vi "Get Main.Parmeters.vi"(0 "Main":string="0", 1 "VI Ref":refnum<vi>, 9 "VariableName":string, 11 "error in (no error)":errorcluster, 12 "Alarm":bool=TRUE) -> (2 "string":string, 3 "Unit":string, 4 "DBL Value":dbl, 6 "Value":string, 10 "Boolean":bool, 13 "Full Results":string[][](array[string]), 14 "Results":string[](array[string]), 15 "error out":errorcluster)   [LabVIEW 2017, in "SQLite.lvclass"]
doc: "get Parmeters.\n2015-11-03 10:59:46\n蒋松\njiangsong@outlook.com"
uses:
  SQLite.lvclass
  SQLiteFileName.ctl
  TabelFullName.ctl
  <userlib>/LabSQL/LabSQL.lvlib
  <userlib>/sushu/sushu.lvlib
panel:
  out "number (0 to 1)":dbl
  out "Select SQL CMD":string
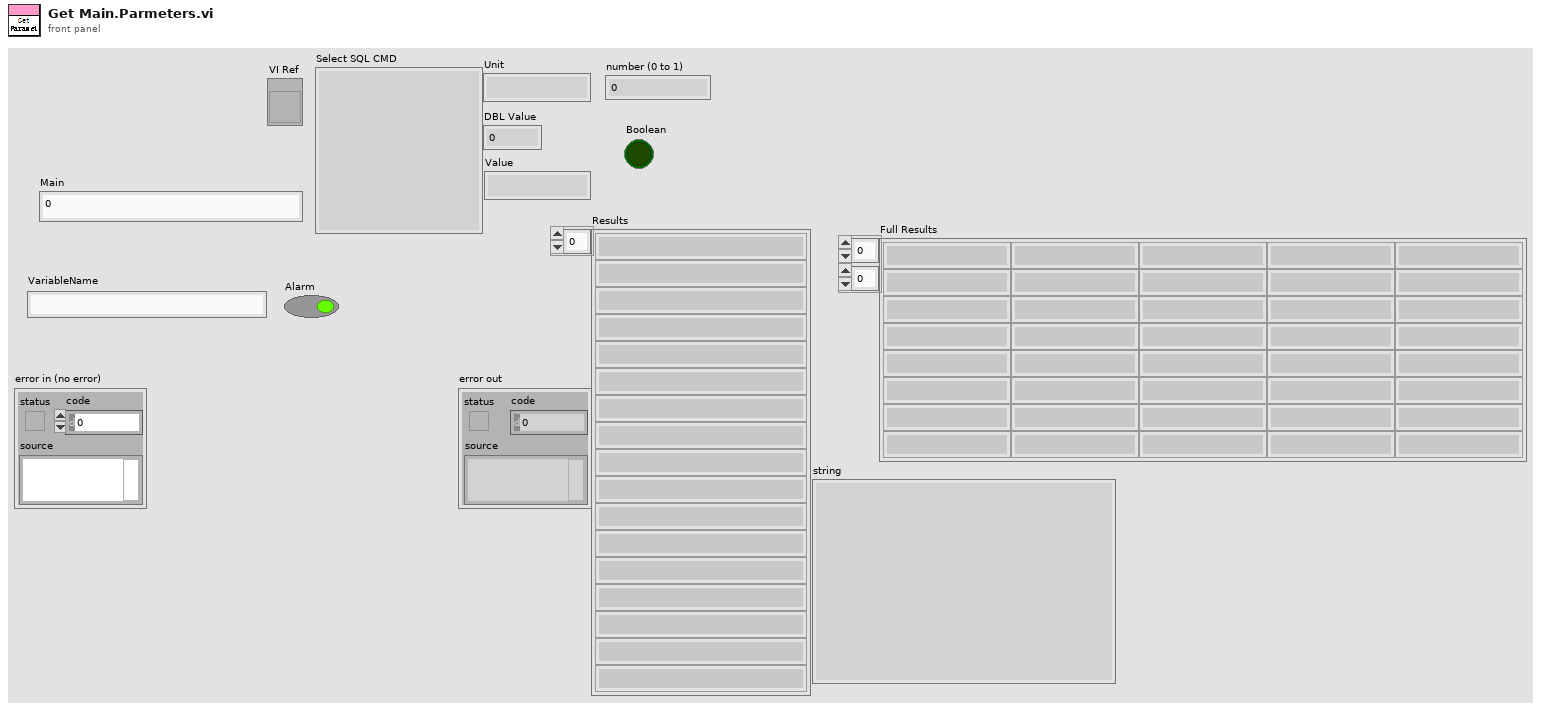
[diagram p1: front panel]
types:
  T1 = enum16{"Initialize", "Read", "Write", "UnInitialize"}
  T2 = typedef "SQLite.lvclass/TabelFullName.ctl" = string
  T3 = typedef "SQLite.lvclass/SQLiteFileName.ctl" = string
  T4 = cluster{"Current VI Reference":refnum<vi>, "Close Panel on Exit?":bool}
  T5 = cluster{"Core":cluster{"Current VI Reference":refnum<vi>, "Close Panel on Exit?":bool}, "VI Name":string}
  T6 = enum16{"Other", "SQL2008", "SQLite", "Access", "MySQL"}
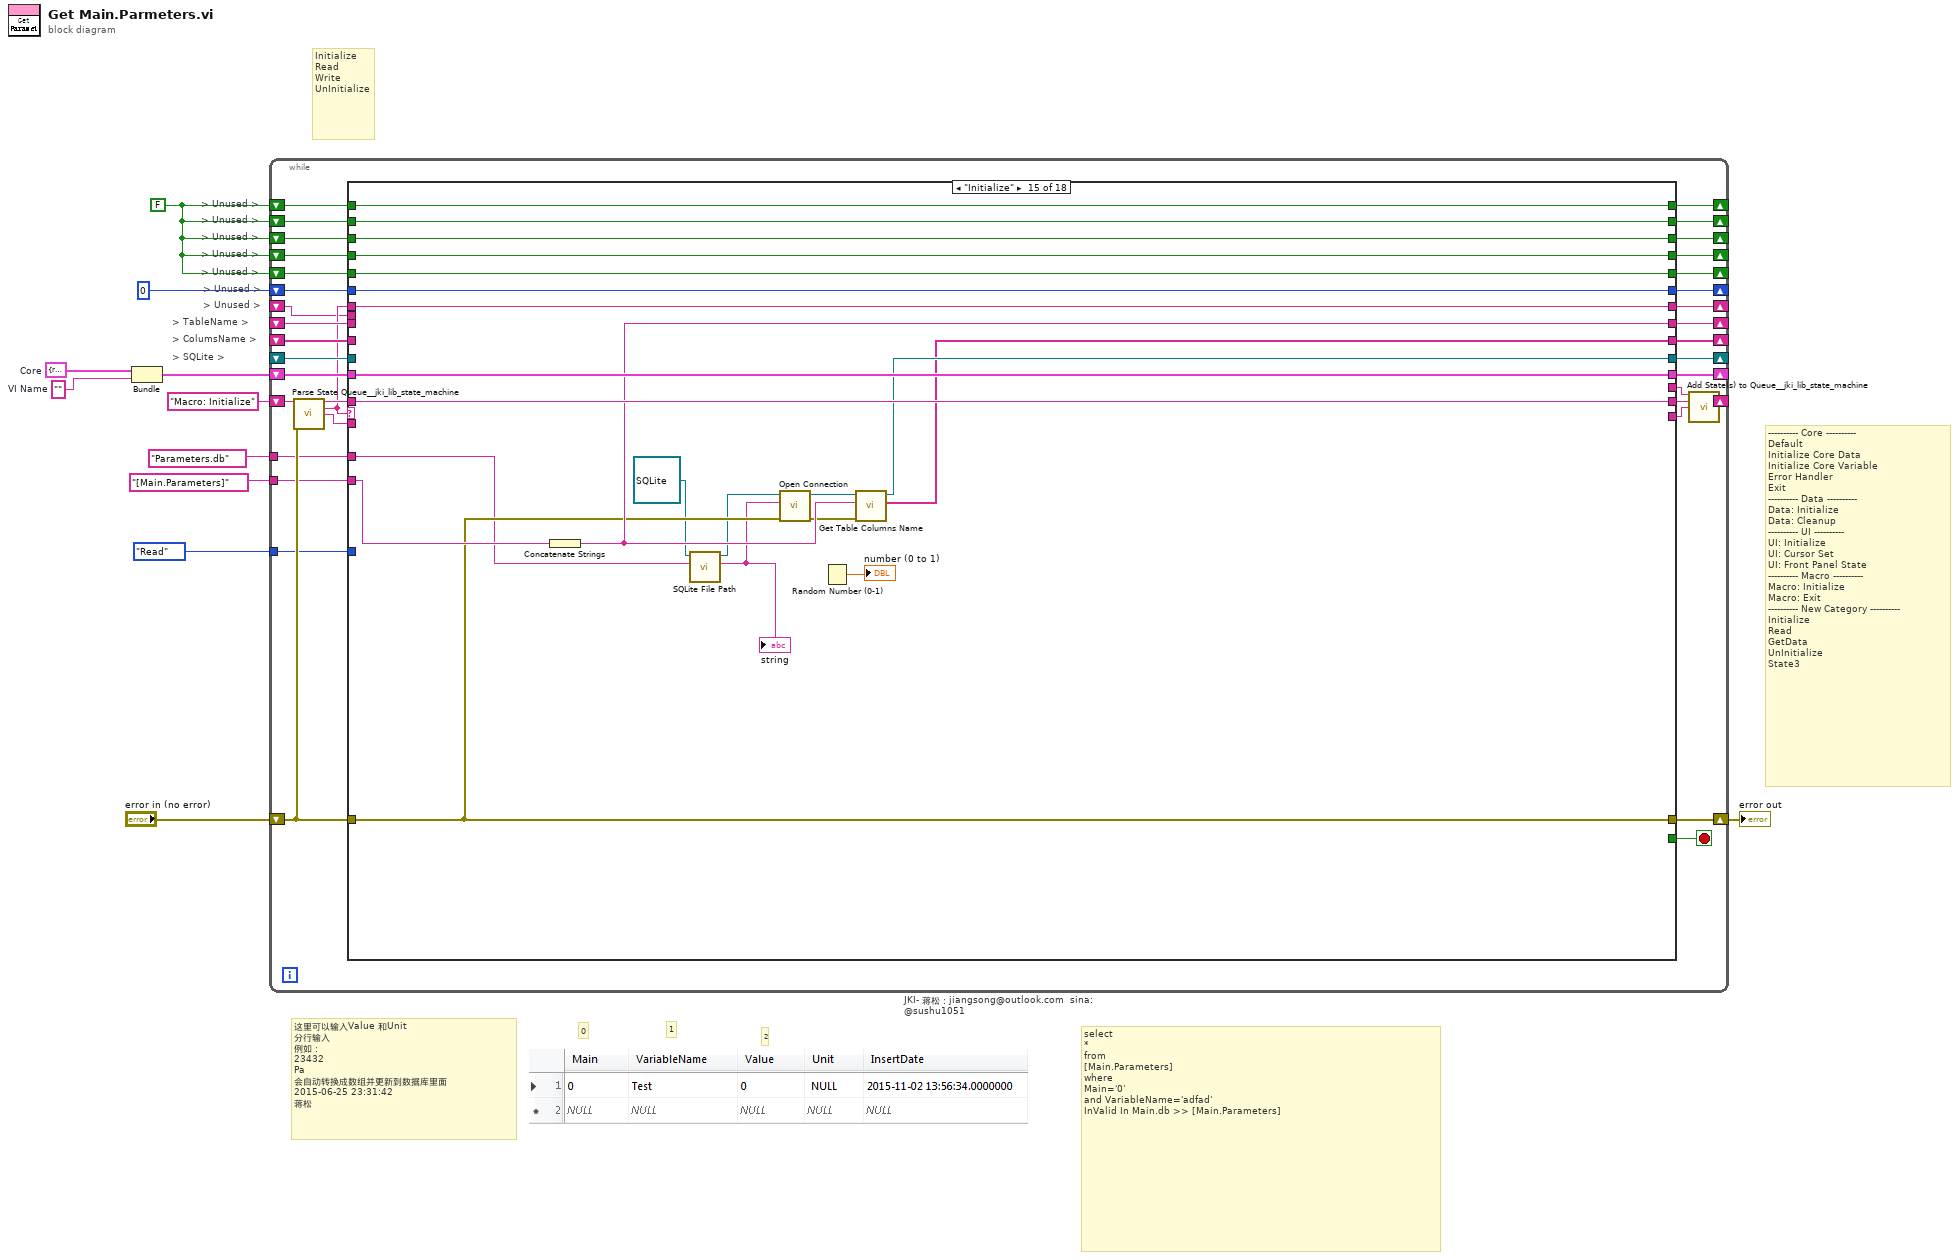
[diagram p0: block diagram]
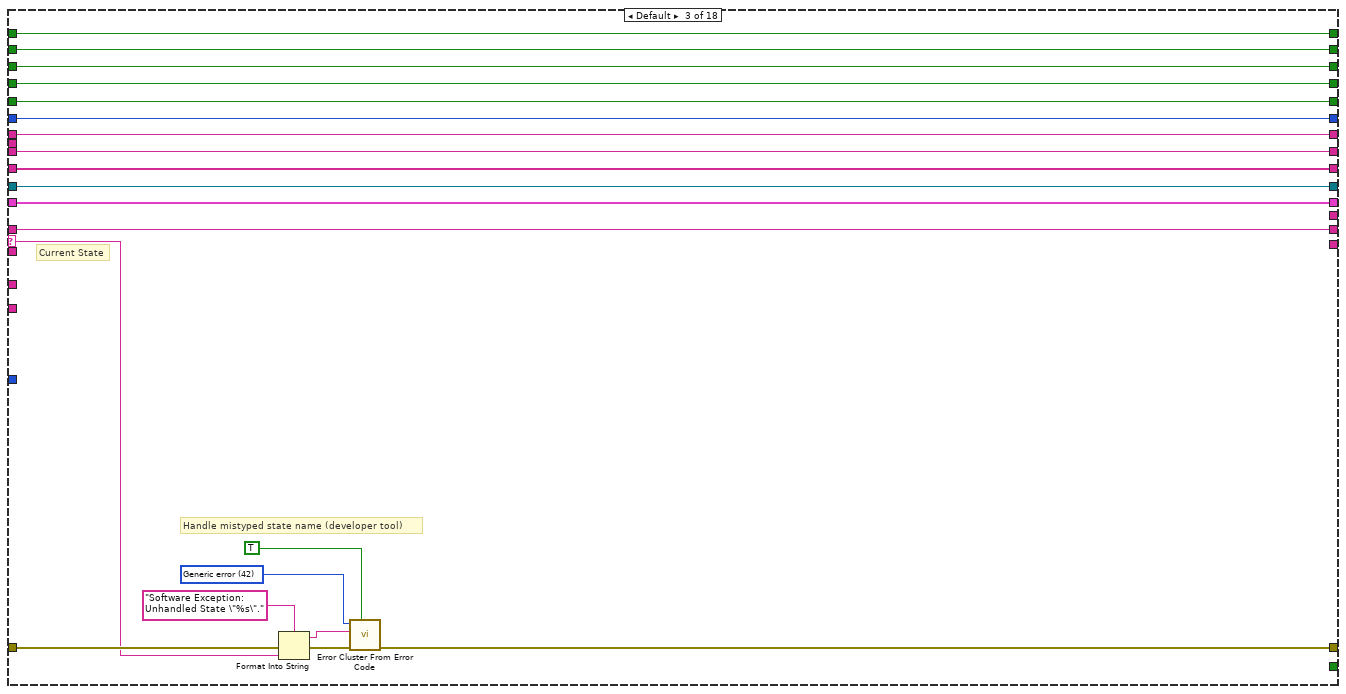
[diagram p4: hidden frame]
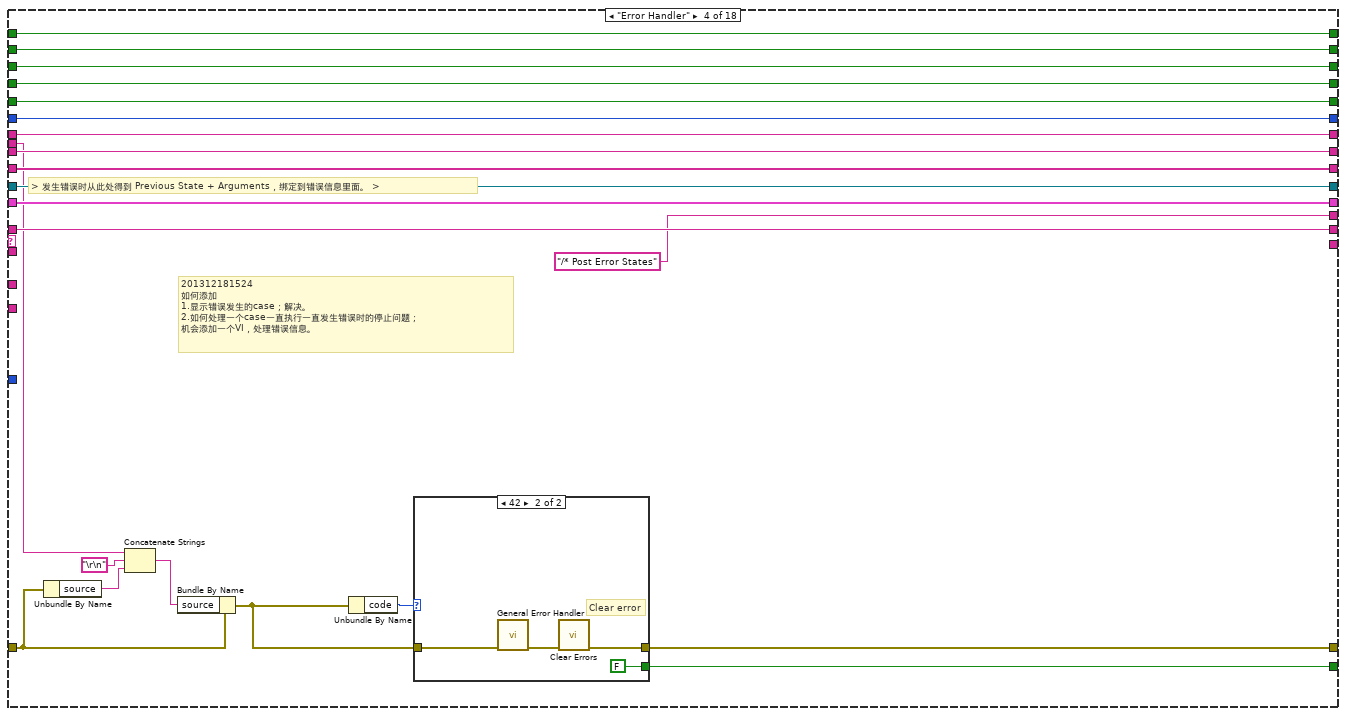
[diagram p5: hidden frame]
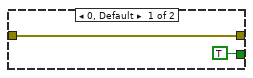
[diagram p6: hidden frame]
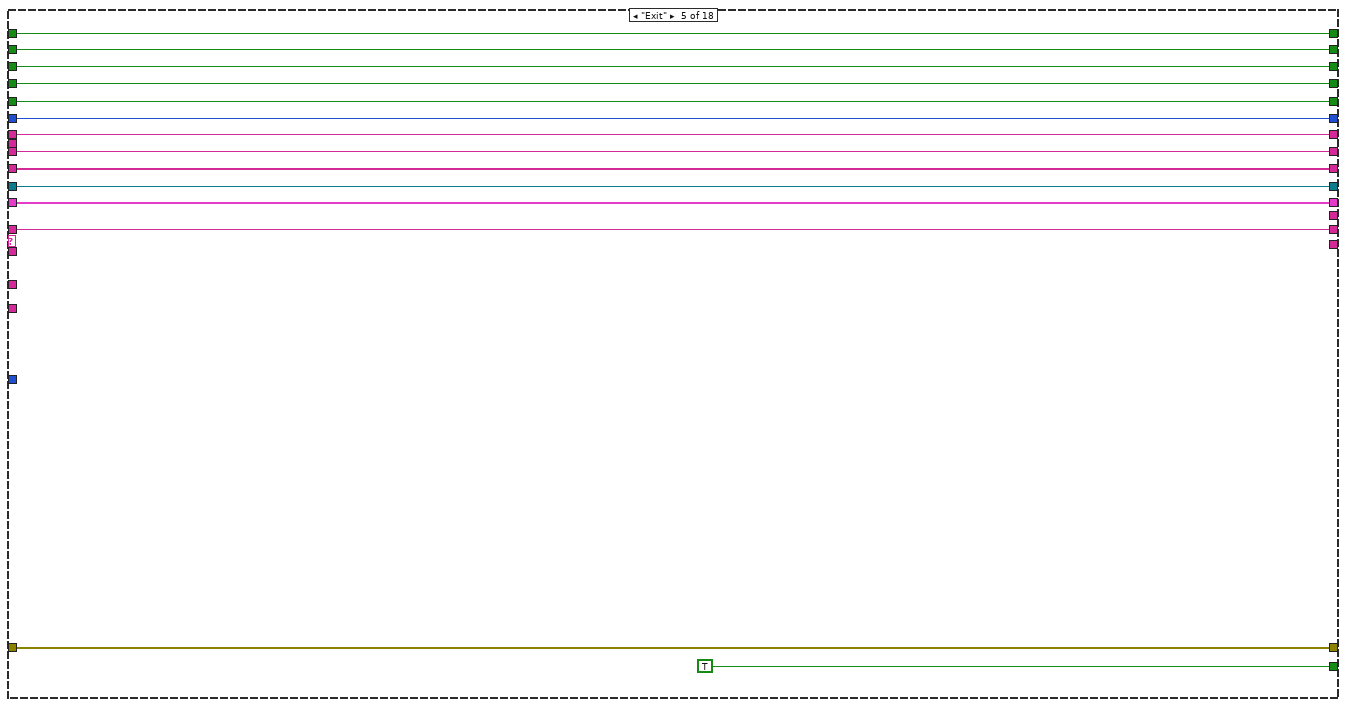
[diagram p7: hidden frame]
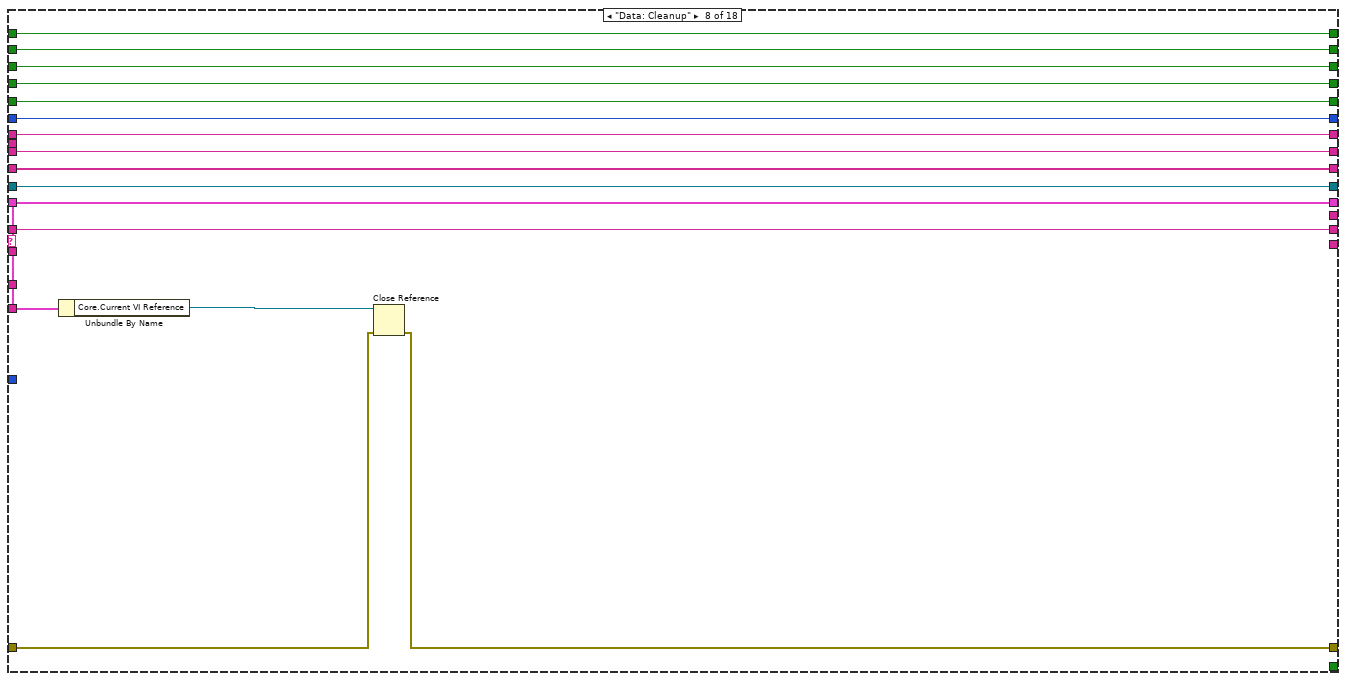
[diagram p10: hidden frame]
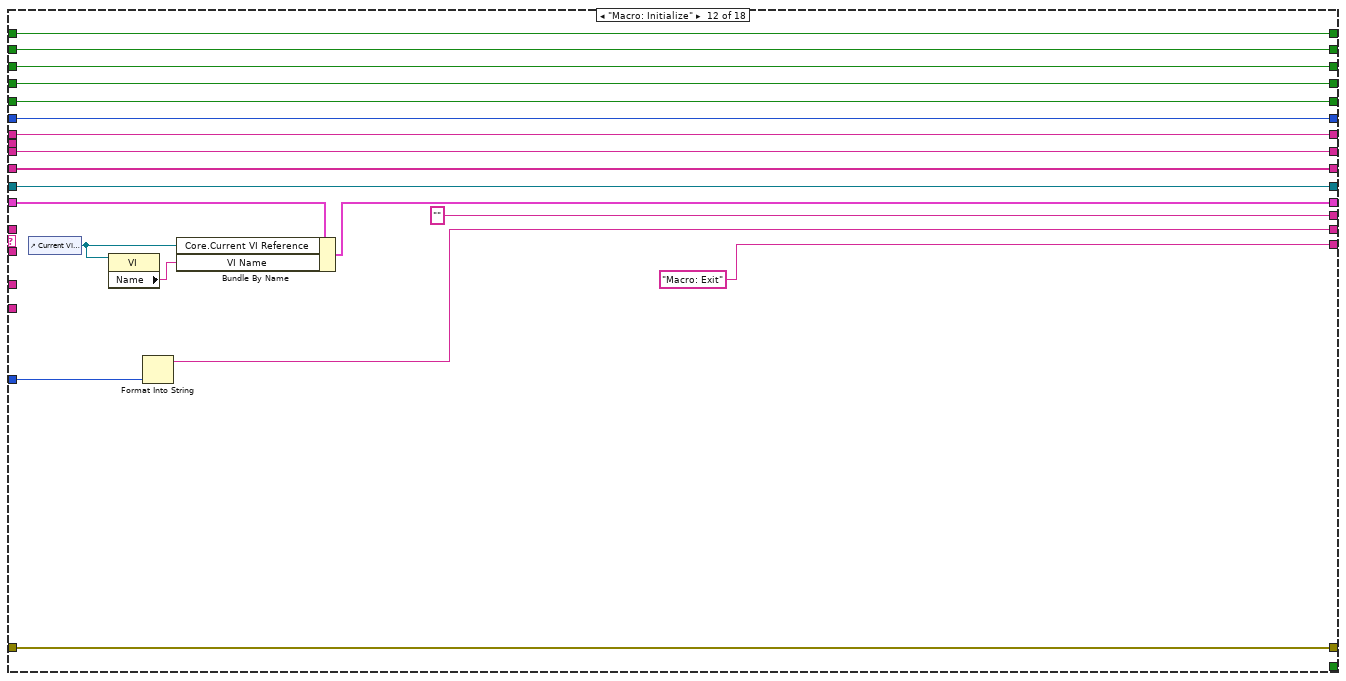
[diagram p14: hidden frame]
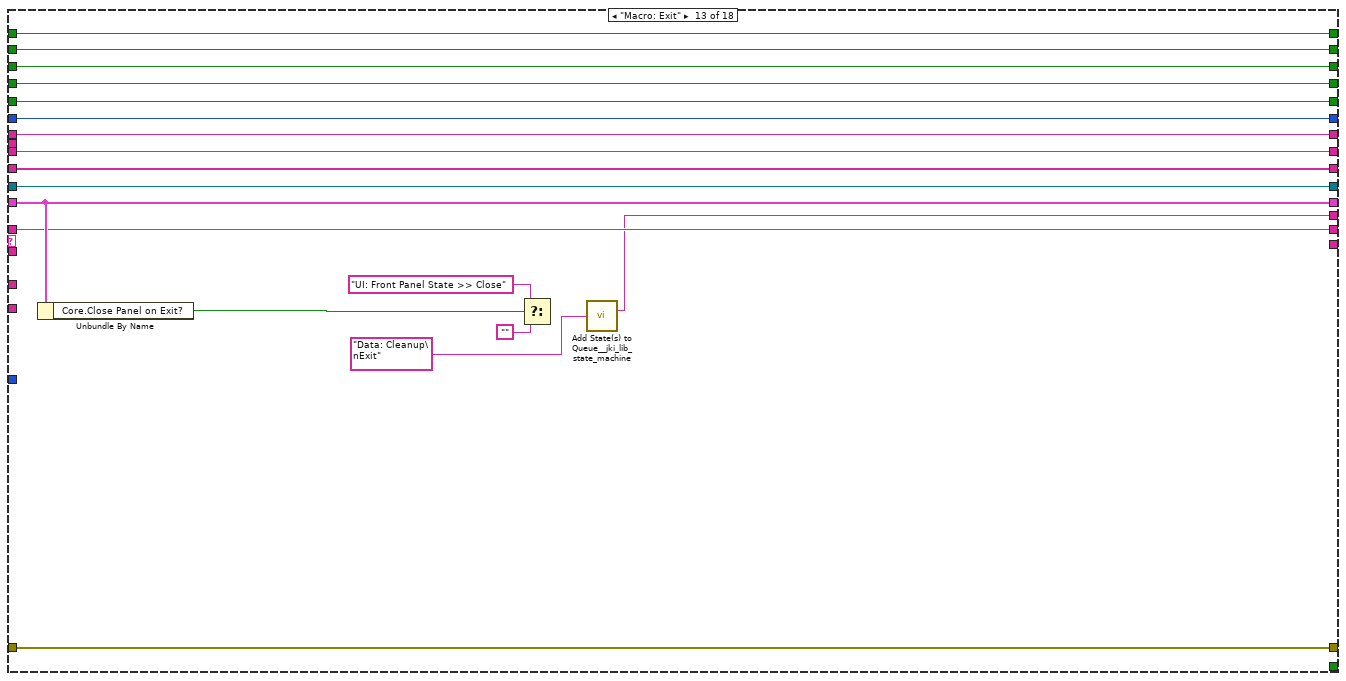
[diagram p15: hidden frame]
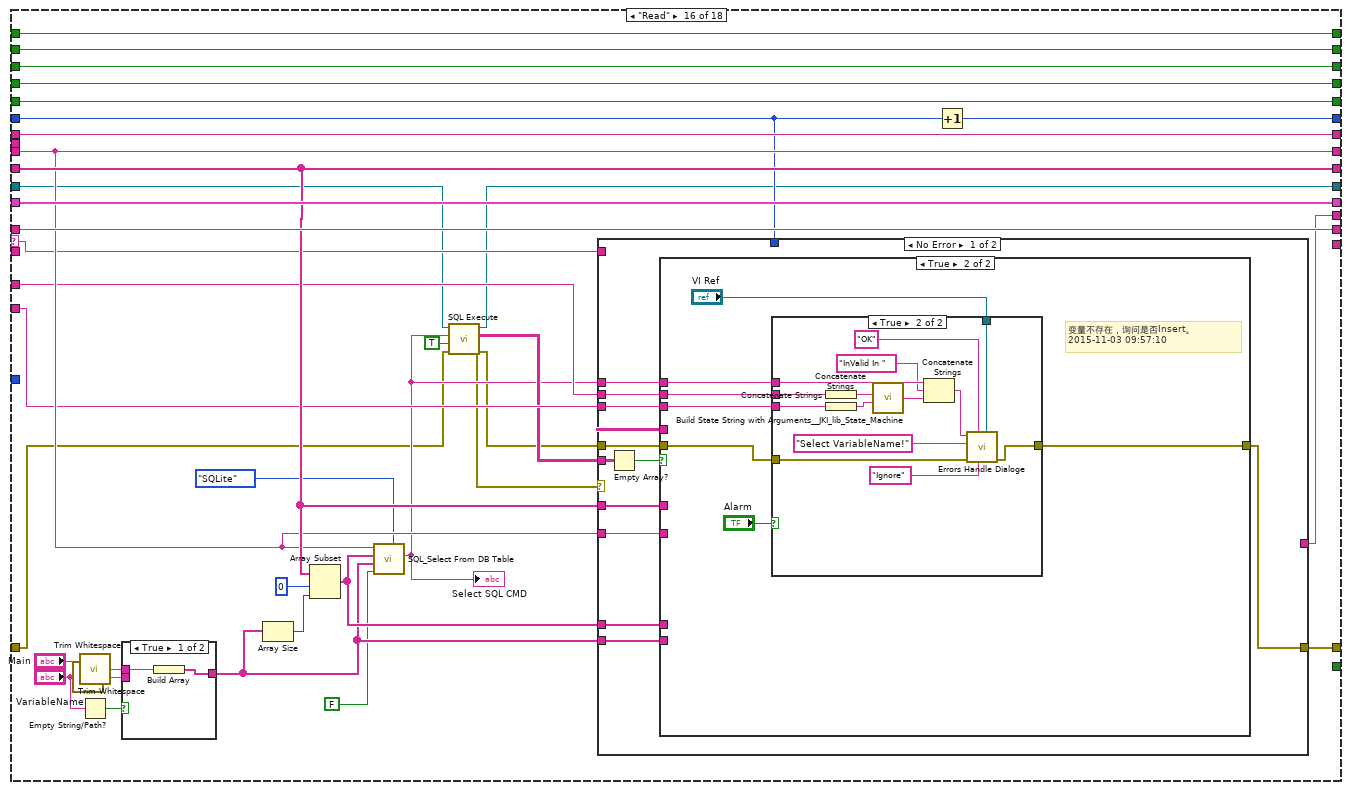
[diagram p17: hidden frame]
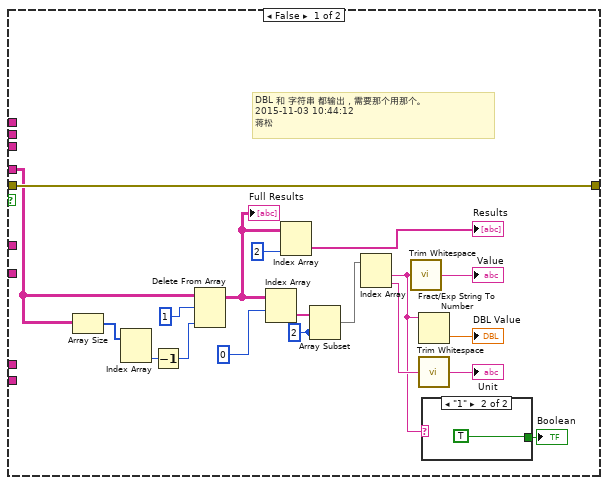
[diagram p18: hidden frame]
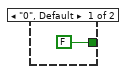
[diagram p19: hidden frame]
diagram:
  w11 = ""  # VI Name
  w10 = T4 {"Current VI Reference"=refnum, "Close Panel on Exit?"=FALSE}  # Core
  w6 = FALSE
  # "Initialize\nRead\nWrite\nUnInitialize"
  # "> Unused >"
  # "> Unused >"
  # "> Unused >"
  # "> Unused >"
  # "> Unused >"
  # "> Unused >"
  # "> SQLite >"
  # "> ColumsName >"
  # "> TableName >"
  # "> Unused >"
  # "---------- Core ----------\nDefault\nInitialize Core Data\nInitialize Core Variable\nError Handler\nExit\n---------- Data ----------\nData: Initialize\nData: Cleanup\n---------- UI ----------\nUI: Initialize\nUI: Cursor Set\nUI: Front Panel State\n---------- Macro ----------\nMacro: Initialize\nMacro: Exit\n---------- New Category ----------\nInitialize\nRead\nGetData\nUnInitialize\nState3"
  # "select\n*\nfrom\n[Main.Parameters]\nwhere\nMain='0'\nand VariableName='adfad'\nInValid In Main.db >> [Main.Parameters]"
  # "2"
  # "1"
  # "0"
  # "这里可以输入Value 和Unit\n分行输入\n例如：\n23432\nPa\n会自动转换成数组并更新到数据库里面\n2015-06-25 23:31:42\n蒋松"
  n1 = Bundle("Core"=w10, "VI Name"=w11) -> (w9:T5)  [unwired: 1 in]
  n2 = while "JKI- 蒋松：jiangsong@outlook.com  sina: @sushu1051" {
    shift-right: [w45] -> w3
    shift-left: "error in (no error)" -> [w43]
    shift-right: [w33] -> _
    shift-left: "Macro: Initialize" -> [w34]
    shift-right: [w40] -> _
    shift-left: _ -> [w42]
    shift-right: [w41] -> _
    shift-left: _ -> [w12]
    shift-right: [w35] -> _
    shift-left: w9 -> [w38]
    shift-right: [w36] -> _
    shift-left: _ -> [w29]
    shift-right: [w37] -> _
    shift-left: _ -> [w39]
    shift-right: [w28] -> _
    shift-left: 0 -> [w27]
    shift-right: [w20] -> _
    shift-left: w6 -> [w18]
    shift-right: [w19] -> _
    shift-left: w6 -> [w17]
    shift-right: [w23] -> _
    shift-left: w6 -> [w24]
    shift-right: [w22] -> _
    shift-left: w6 -> [w21]
    shift-right: [w25] -> _
    shift-left: w6 -> [w26]
    tunnel: T1."Read" ("CMD") -> [w16]
    tunnel: T3 "Parameters.db" ("SQLiteFileName") -> [w15]
    tunnel: T2 "[Main.Parameters]" ("TabelFullName") -> [w14]
    stop <- w44 stop-if-true
    n3 = call <vilib>:"Parse State Queue__jki_lib_state_machine.vi"("State Queue"=w34, "Error In (no error)"=w43) -> ("Remaining States"=w47:string, "Current State"=w13:string, "Arguments"=w46:string)  [unwired: 10 in, 1 out]
    n4 = case shown="\"Initialize\"" w13 {
      selector: w13 -> [_ _ w81 _ _ _ _ _ _ _ _ _ _ _ _ w299 _ _]
      tunnel: w47 -> [w60 w67 w80 w107 w128 w142 w156 w168 w183 w196 w209 _ w242 w259 w286 w321 w405 w420]
      tunnel: w46 -> [_ _ _ _ _ _ _ _ _ _ _ _ _ _ _ _ _ _]
      tunnel: [w59 w73 w82 w101 w130 w144 w158 w170 w185 w198 w211 w231 w249 w262 w271 w300 w393 w406] -> w45
      tunnel: w43 -> [w59 w73 w83 w111 w130 w144 w158 w171 w185 w198 w211 w231 w249 w262 w271 w292 w393 w407]
      tunnel: [w60 w67 w80 w107 w128 w142 w156 w168 w183 w196 w209 w217 w242 w259 w286 w321 w405 w420] -> w32
      tunnel: [_ _ _ w100 TRUE _ _ _ _ _ _ _ _ _ _ _ _ _] -> w44
      tunnel: w13 -> [w58 w72 w93 w115 w135 w148 w161 w176 w189 w202 w215 w234 w252 w265 w285 w301 w395 w419]
      tunnel: w42 -> [w57 w71 w92 w114 w134 w147 w160 w175 w188 w201 w214 w233 w251 w264 _ w305 w404 w418]
      tunnel: [w58 w72 w93 w115 w135 w148 w161 w176 w189 w202 w215 w234 w252 w265 w285 w301 w395 w419] -> w41
      tunnel: [w57 w71 w92 w114 w134 w147 w160 w175 w188 w201 w214 w233 w251 w264 w273 w305 w404 w418] -> w40
      tunnel: w39 -> [w56 w70 w91 w113 w133 w146 w159 w174 w187 w200 w213 w232 w250 w263 _ w306 w403 w417]
      tunnel: w29 -> [w54 w68 w90 w105 w129 w143 w157 w169 w184 w197 w210 w230 w243 w260 _ w296 w402 w409]
      tunnel: w38 -> [w55 w69 w89 w112 w132 w145 w149 w172 w186 w199 w212 w219 w244 w261 w284 w320 w401 w416]
      tunnel: [w56 w70 w91 w113 w133 w146 w159 w174 w187 w200 w213 w232 w250 w263 w274 w306 w403 w417] -> w37
      tunnel: [w54 w68 w90 w105 w129 w143 w157 w169 w184 w197 w210 w230 w243 w260 w275 w294 w402 w408] -> w36
      tunnel: [w55 w69 w89 w112 w132 w145 w149 w172 w186 w199 w212 w218 w244 w261 w284 w320 w401 w416] -> w35
      tunnel: [_ _ _ "/* Post Error States" _ _ _ _ _ _ _ "" w241 _ _ w298 _ _] -> w31
      tunnel: [_ _ _ _ _ _ _ _ _ _ _ "Macro: Exit" _ _ _ _ _ _] -> w30
      tunnel: w27 -> [w53 w66 w79 w104 w127 w141 w155 w167 w182 w195 w208 w229 w240 w258 w283 w297 w400 w415]
      tunnel: [w53 w66 w79 w104 w127 w141 w155 w167 w182 w195 w208 w229 w240 w258 w283 w315 w400 w415] -> w28
      tunnel: w17 -> [w51 w64 w77 w98 w125 w139 w153 w165 w180 w193 w206 w225 w238 w256 w278 w318 w399 w414]
      tunnel: w18 -> [w50 w63 w76 w97 w124 w138 w152 w164 w179 w192 w205 w224 w237 w255 w279 w317 w398 w413]
      tunnel: [w51 w64 w77 w98 w125 w139 w153 w165 w180 w193 w206 w225 w238 w256 w278 w318 w399 w414] -> w19
      tunnel: [w50 w63 w76 w97 w124 w138 w152 w164 w179 w192 w205 w224 w237 w255 w279 w317 w398 w413] -> w20
      tunnel: w21 -> [w49 w62 w75 w96 w123 w137 w151 w163 w178 w191 w204 w223 w236 w254 w280 w316 w397 w412]
      tunnel: w24 -> [w48 w61 w74 w95 w122 w136 w150 w162 w177 w190 w203 w222 w235 w253 w281 w302 w394 w411]
      tunnel: [w49 w62 w75 w96 w123 w137 w151 w163 w178 w191 w204 w223 w236 w254 w280 w316 w397 w412] -> w22
      tunnel: [w48 w61 w74 w95 w122 w136 w150 w162 w177 w190 w203 w222 w235 w253 w281 w302 w394 w411] -> w23
      tunnel: w26 -> [w52 w65 w78 w99 w126 w140 w154 w166 w181 w194 w207 w226 w239 w257 w282 w319 w396 w410]
      tunnel: [w52 w65 w78 w99 w126 w140 w154 w166 w181 w194 w207 w226 w239 w257 w282 w319 w396 w410] -> w25
      tunnel: w16 -> [_ _ _ _ _ _ _ _ _ _ _ w216 _ _ _ _ _ _]
      tunnel: w15 -> [_ _ _ _ _ _ _ _ _ _ _ _ _ _ w267 w303 _ _]
      tunnel: w14 -> [_ _ _ _ _ _ _ _ _ _ _ _ _ _ w276 w304 _ _]
      tunnel: w12 -> [_ _ _ w94 _ _ _ _ _ _ _ _ _ _ _ _ _ _]
      frame "Idle" {
      }
      frame "---------- Core ----------" {
      }
      frame Default {
        w85 = 42 items=["No error", "Argument error", "Memory is full", "Out of zone", "End of file", "File already open", "Generic file I/O error", "File not found", "File permission error", "Disk is full", "Duplicate path", "Too many files open", "System feature not enabled", "Resource file not found", "Cannot add resource", "Resource not found", "Image not found", "Image memory error", "Pen does not exist", "Config type invalid", "Config token not found", "Config parse error", "Config memory error", "Bad external code format", "Bad external code offset", "External code not present", "Null window", "Destroy window error", "Null menu", "Print aborted", "Bad print record", "Print driver error", "Windows error during printing", "Memory error during printing", "Print dialog error", "Generic print error", "Invalid device refnum", "Device not found", "Device parameter error", "Device unit error", "Cannot open device", "Device call aborted", "Generic error", "Cancelled by user", "Object ID too low", "Object ID too high", "Object not in heap", "Unknown heap", "Unknown object (invalid DefProc)", "Unknown object (DefProc not in table)", "Message out of range", "Invalid (null) method", "Unknown message", "Manager call not supported", "Bad address", "Network operation in progress", "Network operation timed out", "Connection is busy", "Network attribute not supported", "Network error", "Address in use", "System out of memory", "Connection aborted", "Connection refused", "Not connected", "Already connected", "Connection closed", "Initialization error (interapplication manager)", "Bad occurrence", "Wait on unbound occurrence handler", "Occurrence queue overflow", "Datalog type conflict", "Unused", "Unrecognized type (interapplication manager)", "Memory corrupt", "Failed to make temporary DLL", "Old CIN version", "Drag socket not found", "Failed to load drop-object", "Failed to register OLE object", "Failed to release OLE object", "Format specifier type mismatch", "Unknown format specifier", "Too few format specifiers", "Too many format specifiers", "Scan failed", "Newer CIN version", "Error converting to variant", "Runtime menu error", "Password tampered", "Variant attribute not found", "Incompatible variant data type", "Event data is not available", "Event Store is not present", "Occurrence is not found", "Event Queue is not created", "Event info is not available", "Refnum passed is NULL", "Error retrieving Class GUID", "Error retrieving CoClass GUID", "Error retrieving TypeLib GUID.", "Bad built application magic bytes.", "Specific driver is different from the specific driver associated with the Logical Name.", "There is no session opened to the class driver.", "Max Error", "MAX - Error with config objects", "MAX - Error loading configuration", "MAX - Group not supported"]
        # "Current State"
        # "Handle mistyped state name (developer tool)"
        n5 = Format Into String(format string="Software Exception: Unhandled State \"%s\"." ("message"), error in=w83, w81) -> (resulting string=w86:string, error out=w87:errorcluster)  [unwired: 1 in]
        n6 = call <vilib>:"Error Cluster From Error Code.vi"("show call chain? (False)"=TRUE, "error in (no error)"=w87, "error message (\"\")"=w86, "error code (0)"=w85) -> ("error out"=w82:errorcluster)  [unwired: 5 in]
      }
      frame "Error Handler" {
        # "> 发生错误时从此处得到 Previous State + Arguments，绑定到错误信息里面。 >"
        # "201312181524\n如何添加\n1.显示错误发生的case；解决。\n2.如何处理一个case一直执行一直发生错误时的停止问题；\n机会添加一个VI，处理错误信息。"
        # "Clear error"
        n7 = Unbundle By Name(w111) -> ("source"=w109:string)
        n8 = Concatenate Strings(w94, "\r\n", w109) -> (w108:string)
        n9 = Bundle By Name(cluster=w111, "source"=w108) -> (w102:errorcluster)
        n10 = Unbundle By Name(w102) -> ("code"=w103:i32)
        n11 = case shown="42" w103 {
          tunnel: [TRUE FALSE] -> w100
          tunnel: w102 -> [w117 w120]
          tunnel: [w117 w118] -> w101
          frame 0, Default {
          }
          frame 42 {
            n12 = call <vilib>:"General Error Handler.vi"("error in (no error)"=w120) -> ("error out"=w119:errorcluster)  [unwired: 10 in, 4 out]
            n13 = call <vilib>:"Clear Errors.vi"("error in (no error)"=w119) -> ("error out"=w118:errorcluster)  [unwired: 5 in, 1 out]
          }
        }
      }
      frame "Exit" {
      }
      frame "---------- Data ----------" {
      }
      frame "Data: Initialize" {
      }
      frame "Data: Cleanup" {
        n14 = Unbundle By Name(w172) -> ("Core.Current VI Reference"=w173:refnum<vi>)
        n15 = Close Reference(reference=w173, error in (no error)=w171) -> (error out=w170:errorcluster)
      }
      frame "---------- UI ----------" {
      }
      frame "UI: Initialize" {
      }
      frame "---------- Macro ----------" {
      }
      frame "Macro: Initialize" {
        n16 = control-ref of="Current VI Reference"() -> (w220:refnum<vi>)
        n17 = property class="VI"(reference=w220) -> ("Name"=w221:string)  [unwired: 1 in, 2 out]
        n18 = Format Into String(w216) -> (resulting string=w217:string)  [unwired: 3 in, 1 out]
        n19 = Bundle By Name(cluster=w219, "Core.Current VI Reference"=w220, "VI Name"=w221) -> (w218:T5)
      }
      frame "Macro: Exit" {
        n20 = Unbundle By Name(w244) -> ("Core.Close Panel on Exit?"=w245:bool)
        n21 = Select(t="UI: Front Panel State >> Close", s=w245, f="") -> ()  [unwired: 1 out]
        n22 = call <vilib>:"Add State(s) to Queue__jki_lib_state_machine.vi"("State(s) at Back (\"\")"="Data: Cleanup\nExit") -> ("States Out"=w241:string)  [unwired: 14 in]
      }
      frame "---------- New Category ----------" {
      }
      frame "Initialize" {
        n23 = Concatenate Strings(w276) -> (w273:string)
        n24 = call "SQLite File Path.vi"("SQLiteFileName"=w267, "SQLite in"=refnum<class "SQLite.lvclass"> refnum ("SQLite.lvclass")) -> ("string"=w270:string, "SQLite out"=w268:refnum<class "SQLite.lvclass">)  [unwired: 7 in, 1 out]
        "string" <- w270
        n25 = call-dynamic "Open Connection.vi"("error in (no error)"=w271, "ConnectionString"=w270, "HostDB in"=w268) -> ("error out"=w272:errorcluster, "HostDB out"=w277:refnum<class "SQLite.lvclass">)  [unwired: 7 in]
        n26 = Random Number (0-1)() -> (number: 0 to 1=→"number (0 to 1)":dbl)
        n27 = call-dynamic "Get Table Columns Name.vi"("error in (no error)"=w272, "TableName"=w273, "HostDB in"=w277) -> ("Table_ColunmsList"=w274:string[], "HostDB out"=w275:refnum<class "SQLite.lvclass">)  [unwired: 3 in, 4 out]
      }
      frame "Read" {
        n28 = call <vilib>:"Trim Whitespace.vi"("string"="VariableName") -> ("trimmed string"=w287:string)  [unwired: 1 in]
        n29 = call <vilib>:"Trim Whitespace.vi"("string"="Main") -> ("trimmed string"=w288:string)  [unwired: 1 in]
        n30 = Empty String/Path?(string/path="VariableName") -> (empty?=w310:bool)
        n31 = case shown="True" w310 {
          tunnel: [w389 w392] -> w309
          tunnel: w288 -> [w388 w391]
          tunnel: w287 -> [_ w390]
          frame True {
            n32 = Build Array(w388) -> (w389:string[])
          }
          frame False {
            n33 = Build Array(w391, w390) -> (w392:string[])
          }
        }
        n34 = Array Size(array=w309) -> (size(s)=w308:i32)
        n35 = Array Subset(array=w306, index=0, length=w308) -> (w314:string[])
        n36 = call <userlib>:"SQL_Select From DB Table.vi"("DB Type"=T6."SQLite", "Check ASCII?"=FALSE, "ColumnsValue"=w309, "ColumnsNameList"=w314, "TableName"=w305) -> ("Select SQL CMD"=w293:string)  [unwired: 6 in]
        "Select SQL CMD" <- w293
        n37 = call-dynamic "SQL Execute.vi"("error in (no error)"=w292, "Return Data (T)"=TRUE, "Command Text"=w293, "HostDB in"=w296) -> ("error out"=w291:errorcluster, "Table Control"=w295:string[][], "HostDB out"=w294:refnum<class "SQLite.lvclass">)  [unwired: 3 in, 2 out]
        n38 = case shown="No Error" w291 {
          selector: w291 -> [_ w380]
          tunnel: w314 -> [w332 _]
          tunnel: w291 -> [w331 w387]
          tunnel: w293 -> [w329 _]
          tunnel: w295 -> [w328 _]
          tunnel: w309 -> [w327 _]
          tunnel: w306 -> [w326 _]
          tunnel: w305 -> [w325 _]
          tunnel: w304 -> [w324 _]
          tunnel: w303 -> [w323 _]
          tunnel: [w322 w386] -> w300
          tunnel: w299 -> [_ w379]
          tunnel: [_ w378] -> w298
          tunnel: w297 -> [_ w377]
          frame No Error {
            n39 = Empty Array?(array=w328) -> (empty?=w330:bool)
            n40 = case shown="True" w330 {
              tunnel: [w351 w359] -> w322
              tunnel: w326 -> [_ _]
              tunnel: w325 -> [_ _]
              tunnel: w327 -> [_ _]
              tunnel: w332 -> [_ _]
              tunnel: w331 -> [w351 w360]
              tunnel: w329 -> [_ w356]
              tunnel: w323 -> [_ w358]
              tunnel: w324 -> [_ w357]
              tunnel: w328 -> [w343 _]
              frame False {
                w344 = 2 ("index")
                # "DBL 和 字符串 都输出，需要那个用那个。\n2015-11-03 10:44:12\n蒋松"
                n41 = Array Size(array=w343) -> (size(s)=w350:i32[])
                n42 = Index Array(array=w350) -> (element #2=w349:i32)  [unwired: 2 in, 1 out]
                n43 = Decrement(x=w349) -> (x-1=w348:i32)
                n44 = Delete From Array(array=w343, length=1 ("disabled index (col)"), index (col)=w348) -> (array with subset deleted=w338:string[][])  [unwired: 1 in, 1 out]
                "Full Results" <- w338
                n45 = Index Array(array=w338, index (row)=0) -> (element=w346:string[])  [unwired: 1 in]
                n46 = Index Array(array=w338, index (col)=2 ("disabled index (col)")) -> (element=→"Results":string[])  [unwired: 1 in]
                n47 = Array Subset(array=w346, index=w344, length=w344) -> (w335:string[])
                n48 = Index Array(array=w335) -> (element #1=w339:string, element #2=w342:string)  [unwired: 2 in]
                n49 = call <vilib>:"Trim Whitespace.vi"("string"=w339) -> ("trimmed string"=→"Value":string)  [unwired: 1 in]
                n50 = Fract/Exp String To Number(string=w339) -> (number=→"DBL Value":dbl)  [unwired: 3 in, 1 out]
                n51 = call <vilib>:"Trim Whitespace.vi"("string"=w342) -> ("trimmed string"=→"Unit":string)  [unwired: 1 in]
                n52 = case shown="\"1\"" w339 {
                  tunnel: [FALSE ("Boolean") TRUE ("Boolean")] -> w340
                  frame "0", Default {
                  }
                  frame "1" {
                  }
                }
                "Boolean" <- w340
              }
              frame True {
                # "变量不存在，询问是否Insert。\n2015-11-03 09:57:10"
                n53 = case shown="True" "Alarm" {
                  tunnel: w360 -> [w361 w375]
                  tunnel: [w361 w374] -> w359
                  tunnel: w358 -> [_ w373]
                  tunnel: w357 -> [_ w372]
                  tunnel: w356 -> [_ w371]
                  tunnel: "VI Ref" -> [_ w362]
                  frame False {
                  }
                  frame True {
                    n54 = Concatenate Strings(w373) -> (w370:string)
                    n55 = Concatenate Strings(w372) -> (w369:string)
                    n56 = call <vilib>:"Build State String with Arguments__JKI_lib_State_Machine.vi"("Arguments (\"\")"=w369, "State"=w370) -> ("State with Arguments"=w367:string)  [unwired: 4 in]
                    n57 = Concatenate Strings(w371, "InValid In " ("Message"), w367) -> (w366:string)
                    n58 = call <userlib>:"Errors Handle Dialoge.vi"("VI Ref"=w362, "Cancel Text"="Ignore", "OK Text"="OK", "error in (no error)"=w375, "Title Text"="Select VariableName!", "Message"=w366) -> ("error out"=w374:errorcluster)  [unwired: 4 in, 1 out]
                  }
                }
              }
            }
          }
          frame Error {
            (unwired) 0
            n59 = call <vilib>:"Clear Errors.vi"("error in (no error)"=w387) -> ("error out"=w386:errorcluster)  [unwired: 5 in, 1 out]
            n60 = Unbundle By Name(w380) -> ("status"=w376:bool)
            n61 = Equal To 0?(x=w377) -> (x = 0?=w384:bool)
            n62 = And(x=w376, y=w384) -> (x .and. y?=w383:bool)
            n63 = call <vilib>:"Add State(s) to Queue__jki_lib_state_machine.vi"("State(s) in Front (\"\")"="Initialize" ("Remaining States"), "State(s) in (\"\")"=w379) -> ("States Out"=w381:string)  [unwired: 13 in]
            n64 = Select(t=w381, s=w383, f="GetData") -> (s? t:f=w378:string)
          }
        }
        n65 = Increment(x=w297) -> (x+1=w315:i32)
      }
      frame "GetData" {
      }
      frame "UnInitialize" {
        n66 = call-dynamic "Close Connection.vi"("error in (no error)"=w407, "HostDB in"=w409) -> ("error out"=w406:errorcluster, "HostDB out"=w408:refnum<class "SQLite.lvclass">)  [unwired: 8 in]
      }
    }
    n67 = call <vilib>:"Add State(s) to Queue__jki_lib_state_machine.vi"("State(s) in Front (\"\")"=w31, "State(s) in (\"\")"=w32, "State(s) at Back (\"\")"=w30) -> ("States Out"=w33:string)  [unwired: 12 in]
  }
  "error out" <- w3
